vi "Set Setting.vi"(7 "Depth":T3 items=["WRITE AREA", "RUNNING AREA", "SAVE AREA"], 8 "error in (no error)":errorcluster, 9 "Setting Data":u8[](array[numeric]), 10 "Target Setting":T1={"Type"=1, "Category"=0, "Item"=0, "Target 1"=0, "Target 2"=0, "Target 3"=0, "Target 4"=0} {"Target 4" format="%.0x"; "Target 3" format="%.0x"; "Target 2" format="%.0x"; "Target 1" format="%.0x"; "Item" format="%.0x"; "Category" format="%.0x"; "Type" items=["ENVIRONMENT"=1, "COMMON MEASUREMENT"=2, "PROGRAM 0"=16, "PROGRAM 1"=17, "PROGRAM 2"=18, "PROGRAM 3"=19, "PROGRAM 4"=20, "PROGRAM 5"=21, "PROGRAM 6"=22, "PROGRAM 7"=23, "PROGRAM 8"=24, "PROGRAM 9"=25, "PROGRAM 10"=26, "PROGRAM 11"=27, "PROGRAM 12"=28, "PROGRAM 13"=29, "PROGRAM 14"=30, "PROGRAM 15"=31]}, 11 "Device ID (0)":i32) -> (0 "error out":errorcluster, 2 "Setting Error":u32 format="%.0x", 3 "Device ID out":i32)   [LabVIEW 2015, in "KEYENCE LJ-X8000A.lvlib"]
doc: "This function sends the setting for the specified item to the controller."
uses:
  KEYENCE LJ-X8000A.lvlib
  Constants/Setting Depth.ctl
  Clusters/Target Setting.ctl
  Constants/Setting Type.ctl
panel:
  # "(c) 2019 KEYENCE CORPORATION.  ALL RIGHTS RESERVED."
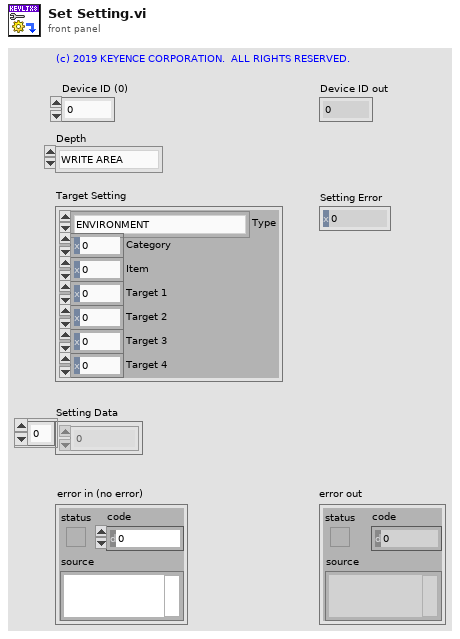
[diagram p1: front panel]
types:
  T1 = typedef "KEYENCE LJ-X8000A.lvlib/Target Setting.ctl" = cluster{"Type":T2, "Category":u8, "Item":u8, "Target 1":u8, "Target 2":u8, "Target 3":u8, "Target 4":u8}
  T2 = typedef "KEYENCE LJ-X8000A.lvlib/Setting Type.ctl" = u8
  T3 = typedef "KEYENCE LJ-X8000A.lvlib/Setting Depth.ctl" = u8
  T4 = cluster{"Type":T2, "Category":u8, "Item":u8, "reserve":u8, "Target 1":u8, "Target 2":u8, "Target 3":u8, "Target 4":u8}
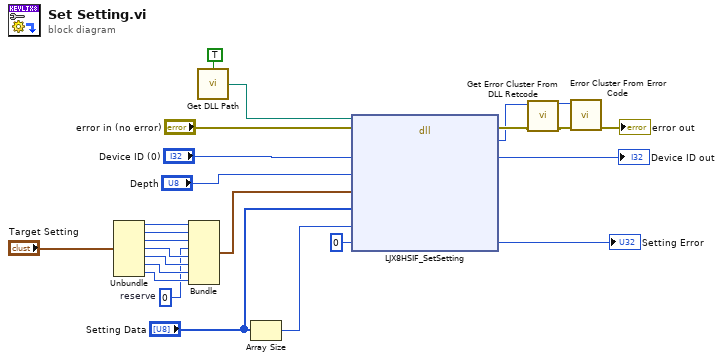
[diagram p0: block diagram]
diagram:
  w15 = u8 0  # reserve
  n1 = Unbundle("Target Setting") -> ("Type"=w22:T2, "Category"=w21:u8, "Item"=w20:u8, "Target 1"=w19:u8, "Target 2"=w18:u8, "Target 3"=w17:u8, "Target 4"=w16:u8)
  n2 = Bundle("Type"=w22, "Category"=w21, "Item"=w20, "reserve"=w15, "Target 1"=w19, "Target 2"=w18, "Target 3"=w17, "Target 4"=w16) -> (w14:T4)  [unwired: 1 in]
  n3 = call "Get DLL Path.vi"("isWrapperDLL (False)"=TRUE) -> ("DLL Path"=w7:path)  [unwired: 2 in]
  n4 = Array Size(array="Setting Data") -> (size(s)=w12:i32)
  n5 = dll-call lib="C:/Program Files (x86)/National Instruments/LabVIEW 2018/instr.lib/KEYENCE LJ-X8000/LJX8_HighSpeedWrapper.*" fn="LJX8HSIF_SetSetting"(path in=w7, error in="error in (no error)", "lDeviceId"="Device ID (0)", "byDepth"="Depth", "pTargetSetting"=w14, "pData"="Setting Data", "dwDataSize"=w12, "pdwError"=u32 0) -> (error out=w5:errorcluster, "lRetCode"=w4:i32, "lDeviceId"=→"Device ID out":i32, "pdwError"=→"Setting Error":u32)  [unwired: 5 in, 1 out]
  n6 = call "Get Error Cluster From DLL Retcode.vi"("error in (no error)"=w5, "DLL Return Code"=w4) -> ("error out"=w6:errorcluster, "VI Error Code"=w1:i32)  [unwired: 8 in]
  n7 = call <vilib>:"Error Cluster From Error Code.vi"("error in (no error)"=w6, "error code (0)"=w1) -> ("error out"=→"error out":errorcluster)  [unwired: 7 in]
